vi "Read Graph.vi"(8 "error in (no error)":errorcluster, 11 "PLBB in":refnum<class "Test Device.lvclass">) -> (0 "error out":errorcluster, 2 "graph":sgl[](array[numeric]), 3 "PLBB out":refnum<class "Test Device.lvclass">)   [LabVIEW 2015, in "Test Device.lvclass"]
uses:
  Test Device.lvclass
  <vilib>/plasmapper/PL Modbus Client/PL Modbus Client.lvclass
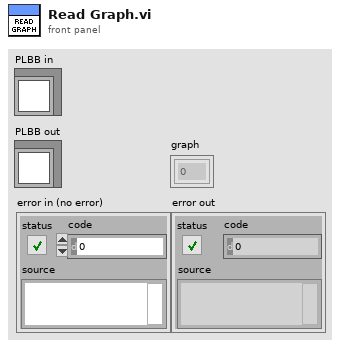
[diagram p1: front panel]
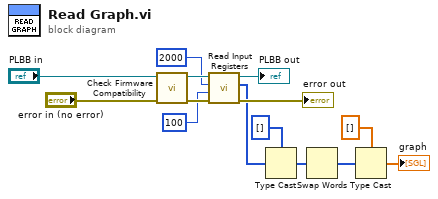
[diagram p0: block diagram]
diagram:
  n1 = call-dynamic "Check Firmware Compatibility.vi"("error in (no error)"="error in (no error)", "TD in"="PLBB in") -> ("error out"=w12:errorcluster, "TD out"=w11:refnum<class "Test Device.lvclass">)  [unwired: 8 in]
  n2 = call <vilib>:"Read Input Registers.vi"("error in (no error)"=w12, "number of input registers"=u16 100, "address"=u16 2000, "MODBUS in"=w11) -> ("error out"=→"error out":errorcluster, "values"=w6:u16[], "MODBUS out"=→"PLBB out":refnum<class "Test Device.lvclass">)  [unwired: 5 in]
  n3 = Type Cast(type=u32[] [] ("graph"), x=w6) -> (*(type *) &x=w4:u32[])
  n4 = Swap Words(1:w4) -> (0:w2:u32[])
  n5 = Type Cast(type=sgl[] [] ("graph"), x=w2) -> (*(type *) &x=→"graph":sgl[])
